vi "motor_test_simple_controller.vi"() -> ()   [LabVIEW 2019]
uses:
  motors_axis_enum_typedef.ctl
  <vilib>/Instr/_visa.llb/VISA Configure Serial Port (Instr).vi
panel:
  in  "VISA resource name":refnum<visa-resource-name>
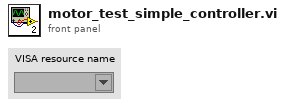
[diagram p1: front panel]
types:
  T1 = typedef "motors_axis_enum_typedef.ctl" = enum16{"Polarizer 1", "Polarizer 2", "Sample", "Stage"}
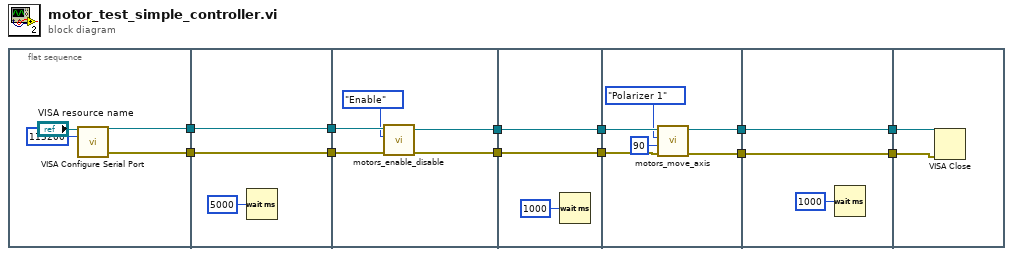
[diagram p0: block diagram]
diagram:
  n1 = flat-sequence {
    tunnel: [w14] -> w12
    tunnel: [w13] -> w10
    tunnel: w12 -> [w18]
    tunnel: [w18] -> w11
    tunnel: w10 -> [w17]
    tunnel: [w17] -> w9
    tunnel: w11 -> [w24]
    tunnel: w9 -> [w23]
    tunnel: [w21] -> w8
    tunnel: [w20] -> w5
    tunnel: w8 -> [w26]
    tunnel: [w26] -> w7
    tunnel: [w25] -> w6
    tunnel: w5 -> [w25]
    tunnel: w7 -> [w33]
    tunnel: w6 -> [w32]
    tunnel: [w29] -> w3
    tunnel: [w28] -> w1
    tunnel: [w35] -> w4
    tunnel: w3 -> [w35]
    tunnel: [w34] -> w2
    tunnel: w1 -> [w34]
    tunnel: w4 -> [w38]
    tunnel: w2 -> [w37]
    frame #0 {
      n2 = call-poly "VISA Configure Serial Port"("VISA resource name"="VISA resource name", "baud rate (9600)"=u32 115200) -> ("VISA resource name out"=w14:refnum<visa-resource-name>, "error out"=w13:errorcluster)  [unwired: 12 in]
    }
    frame #1 {
      n3 = Wait (ms)(milliseconds to wait=u32 5000) -> ()  [unwired: 1 out]
    }
    frame #2 {
      n4 = call "motors_enable_disable.vi"("Error In"=w23, "Status"=enum16{"Disable", "Enable"}."Enable", "VISA resource name"=w24) -> ("Error Out"=w20:errorcluster, "VISA resource name out"=w21:refnum<visa-resource-name>)  [unwired: 7 in]
    }
    frame #3 {
      n5 = Wait (ms)(milliseconds to wait=u32 1000) -> ()  [unwired: 1 out]
    }
    frame #4 {
      n6 = call "motors_move_axis.vi"("Error In"=w32, "Position"=u16 90, "Axis"=motors_axis_enum_typedef."Polarizer 1", "VISA resource name"=w33) -> ("Error Out"=w28:errorcluster, "VISA resource name out"=w29:refnum<visa-resource-name>)  [unwired: 6 in]
    }
    frame #5 {
      n7 = Wait (ms)(milliseconds to wait=u32 1000) -> ()  [unwired: 1 out]
    }
    frame #6 {
      n8 = VISA Close(VISA resource name=w38, error in (no error)=w37) -> ()  [unwired: 1 out]
    }
  }
